vi "Pre Launch Init.vi"(11 "Assert Service in":refnum<class "Assert Service.lvclass">) -> (0 "error out":errorcluster, 3 "Assert Service out":refnum<class "Assert Service.lvclass">)   [LabVIEW 2016, in "Assert Service.lvlib" / "Assert Service.lvclass"]
doc: "(<B>Filename</B>: Actor Framework.lvlib:Actor.lvclass:Pre Launch Init.vi)\n\nDefines behavior that occurs after the Launch Nested Actor method is invoked but before the actor's Actor Core method begins running.\n\nBy default, this method does nothing. A descendant class may override it to define behavior."
uses:
  Assert Service.lvclass
  Assert Service.lvclass/Assert Service.ctl
  Service Actions/UDP Listener/UDP Listener.lvclass
  C:/Users/ukhornp/Documents/Work/Projects/actor_assert_api/Core/Assert Service/Service Actions/Service Action Base.lvclass
  Service Actions/UDP Listener/UDP Listener.lvclass/UDP Listener.ctl
  <vilib>/ActorFramework/Message Enqueuer/Message Enqueuer.lvclass
  Base UI Actor/Base UI Actor/Base UI Actor.lvclass
  Service Actions/Service Action Base.lvclass
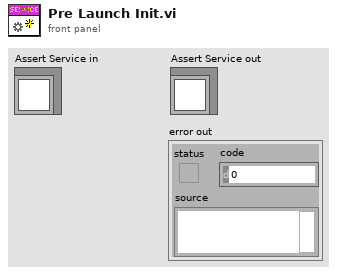
[diagram p1: front panel]
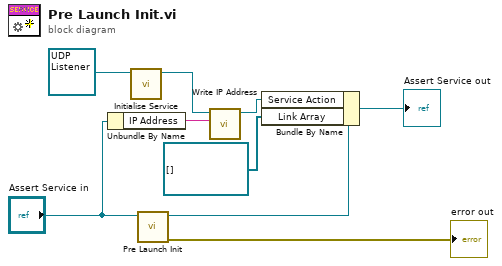
[diagram p0: block diagram]
diagram:
  n1 = Unbundle By Name("Assert Service in") -> ("IP Address"=w5:string)
  n2 = call "Initialise Service.vi"("Service Action Base in"=refnum<class "UDP Listener.lvclass"> refnum ("Assert API Components.lvlib:Assert Service.lvlib:UDP Listener.lvclass")) -> ("Service Action Base out"=w2:refnum<class "UDP Listener.lvclass">)  [unwired: 10 in]
  n3 = call-parent "Pre Launch Init.vi"("Base UI Actor in"="Assert Service in") -> ("error out"=→"error out":errorcluster, "Base UI Actor out"=w8:refnum<class "Assert Service.lvclass">)  [unwired: 9 in]
  n4 = call "Write IP Address.vi"("IP Address"=w5, "UDP Listener in"=w2) -> ("UDP Listener out"=w3:refnum<class "UDP Listener.lvclass">)  [unwired: 9 in]
  n5 = Bundle By Name(cluster=w8, "Service Action"=w3, "Link Array"=refnum<class "Message Enqueuer.lvclass">[] []) -> (→"Assert Service out":refnum<class "Assert Service.lvclass">)
